vi "ex4.vi"() -> ()   [LabVIEW 2022 SP3]
panel:
  out "Out":dbl
  in  "In":dbl
  in  "Typ konwersji":enum16{"C -> F", "F -> C"}(ring)
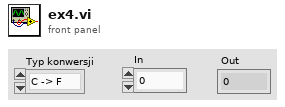
[diagram p1: front panel]
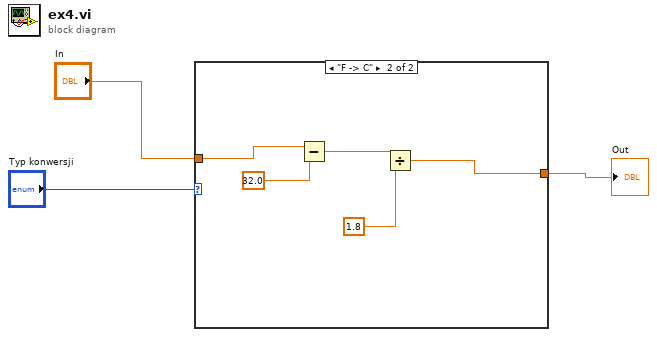
[diagram p0: block diagram]
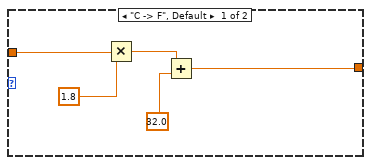
[diagram p2: hidden frame]
diagram:
  n1 = case shown="\"F -> C\"" "Typ konwersji" {
    tunnel: [w5 w10] -> w2
    tunnel: "In" -> [w4 w9]
    frame "C -> F", Default {
      n2 = Multiply(x=w4, y=1.8) -> (x*y=w7:dbl)
      n3 = Add(x=w7, y=32.0) -> (x+y=w5:dbl)
    }
    frame "F -> C" {
      n4 = Subtract(x=w9, y=32.0) -> (x-y=w12:dbl)
      n5 = Divide(x=w12, y=1.8) -> (x/y=w10:dbl)
    }
  }
  "Out" <- w2
